vi "Modbus send and receive.vi"(6 "Modbus telegram":string, 7 "COM port":refnum<visa-resource-name>) -> (0 "Comms error":errorcluster, 1 "Device response":u8[](array[numeric]) format="%02x", 2 "Modbus exception code":T1 items=["None"=0, "Invalid function request"=1, "Invalid Modbus register address"=2, "Invalid / unauthorised data value"=3, "Device failure"=4, "Request accepted, wait"=5, "Drive busy"=6, "Request rejected"=7, "Memory parity error"=8, "Gateway path unavailable"=10, "Device failed to respond"=11], 3 "Checksum ok":bool)   [LabVIEW 2020]
doc: "Modbus RTU for Invertek drives. Paul Nathan 19-JUN-2022."
uses:
  ctls/Exception codes.ctl
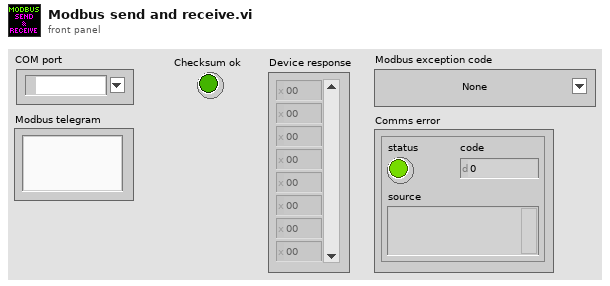
[diagram p1: front panel]
types:
  T1 = typedef "Exception codes.ctl" = u8
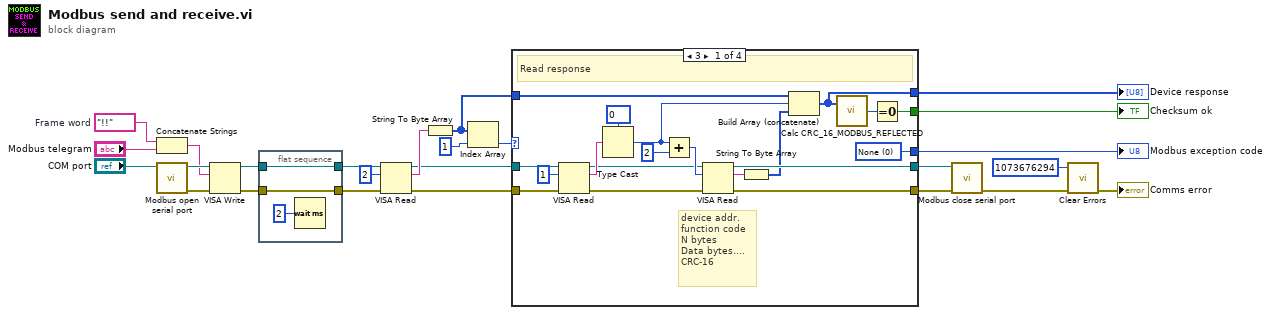
[diagram p0: block diagram]
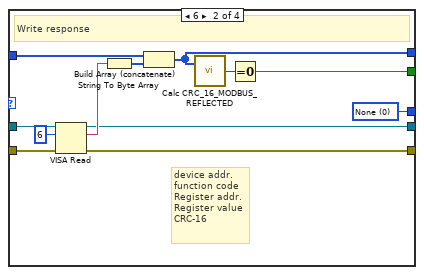
[diagram p2: hidden frame]
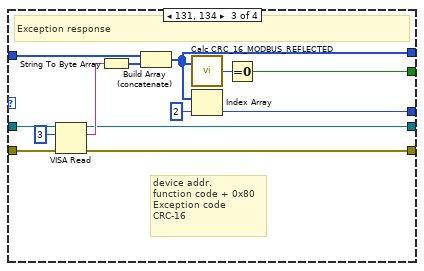
[diagram p3: hidden frame]
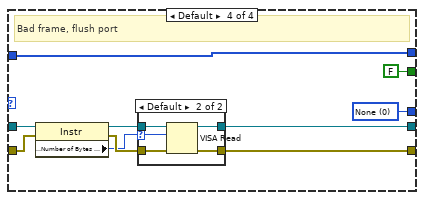
[diagram p4: hidden frame]
diagram:
  w1 = "!!"  # Frame word
  n1 = Concatenate Strings(w1, "Modbus telegram") -> (w2:string)
  n2 = call "Modbus open serial port.vi"("VISA resource name"="COM port") -> ("Error out"=w24:errorcluster, "VISA resource name out"=w25:refnum<visa-resource-name>)  [unwired: 9 in]
  n3 = VISA Write(VISA resource name=w25, write buffer=w2, error in (no error)=w24) -> (VISA resource name out=w7:refnum<visa-resource-name>, error out=w6:errorcluster)  [unwired: 1 out]
  n4 = flat-sequence {
    tunnel: w7 -> [w28]
    tunnel: w6 -> [w27]
    tunnel: [w28] -> w5
    tunnel: [w27] -> w4
    frame #0 {
      n5 = Wait (ms)(milliseconds to wait=u32 2) -> ()  [unwired: 1 out]
    }
  }
  n6 = VISA Read(VISA resource name=w5, byte count=u32 2, error in (no error)=w4) -> (VISA resource name out=w21:refnum<visa-resource-name>, read buffer=w22:string, error out=w20:errorcluster)  [unwired: 1 out]
  n7 = String To Byte Array(string=w22) -> (unsigned byte array=w16:u8[])
  n8 = Index Array(array=w16, index=1) -> (element=w17:u8)
  n9 = case shown="3" w17 {
    tunnel: w21 -> [w47 w59 w68 w82]
    tunnel: w20 -> [w46 w58 w67 w81]
    tunnel: [w37 w53 w64 w78] -> w19
    tunnel: [w33 w50 w65 FALSE] -> w13
    tunnel: [w32 w49 w62 w76] -> w12
    tunnel: w16 -> [w31 w56 w66 w76]
    tunnel: [w30 w52 w63 w77] -> w15
    tunnel: [w29 w48 w60 w74] -> w14
    frame 3 {
      w29 = T1 0 items=["None"=0, "Invalid request"=1, "Invalid Modbus register"=2, "Register value out of range"=3, "Device failure"=4, "Request accepted, wait"=5, "Drive busy"=6, "Request rejected"=7, "Memory parity error"=8, "Gateway path unavailable"=10, "Device failed to respond"=11] ("Modbus exception code")
      # "device addr.\nfunction code\nN bytes\nData bytes....\nCRC-16"
      # "Read response"
      n10 = VISA Read(VISA resource name=w47, byte count=u32 1, error in (no error)=w46) -> (VISA resource name out=w40:refnum<visa-resource-name>, read buffer=w44:string, error out=w39:errorcluster)  [unwired: 1 out]
      n11 = Type Cast(type=u8 0 ("index"), x=w44) -> (*(type *) &x=w36:u8)
      n12 = Add(x=w36, y=u32 2) -> (x+y=w41:u32)
      n13 = VISA Read(VISA resource name=w40, byte count=w41, error in (no error)=w39) -> (VISA resource name out=w37:refnum<visa-resource-name>, read buffer=w38:string, error out=w30:errorcluster)  [unwired: 1 out]
      n14 = String To Byte Array(string=w38) -> (unsigned byte array=w35:u8[])
      n15 = Build Array (concatenate)(w31, w36, w35) -> (w32:u8[])
      n16 = call "Calc CRC_16_MODBUS_REFLECTED.vi"("Data bytes"=w32) -> ("CRC_16-MODBUS"=w34:u16)  [unwired: 1 in]
      n17 = Equal To 0?(x=w34) -> (x = 0?=w33:bool)
    }
    frame 6 {
      w48 = T1 0 items=["None"=0, "Invalid request"=1, "Invalid Modbus register"=2, "Register value out of range"=3, "Device failure"=4, "Request accepted, wait"=5, "Drive busy"=6, "Request rejected"=7, "Memory parity error"=8, "Gateway path unavailable"=10, "Device failed to respond"=11] ("Modbus exception code")
      # "device addr.\nfunction code\nRegister addr.\nRegister value\nCRC-16"
      # "Write response"
      n18 = VISA Read(VISA resource name=w59, byte count=u32 6, error in (no error)=w58) -> (VISA resource name out=w53:refnum<visa-resource-name>, read buffer=w55:string, error out=w52:errorcluster)  [unwired: 1 out]
      n19 = String To Byte Array(string=w55) -> (unsigned byte array=w54:u8[])
      n20 = Build Array (concatenate)(w56, w54) -> (w49:u8[])
      n21 = call "Calc CRC_16_MODBUS_REFLECTED.vi"("Data bytes"=w49) -> ("CRC_16-MODBUS"=w51:u16)  [unwired: 1 in]
      n22 = Equal To 0?(x=w51) -> (x = 0?=w50:bool)
    }
    frame 131, 134 {
      # "device addr.\nfunction code + 0x80\nException code\nCRC-16"
      # "Exception response"
      n23 = VISA Read(VISA resource name=w68, byte count=u32 3, error in (no error)=w67) -> (VISA resource name out=w64:refnum<visa-resource-name>, read buffer=w72:string, error out=w63:errorcluster)  [unwired: 1 out]
      n24 = String To Byte Array(string=w72) -> (unsigned byte array=w71:u8[])
      n25 = Build Array (concatenate)(w66, w71) -> (w62:u8[])
      n26 = call "Calc CRC_16_MODBUS_REFLECTED.vi"("Data bytes"=w62) -> ("CRC_16-MODBUS"=w70:u16)  [unwired: 1 in]
      n27 = Index Array(array=w62, index=2) -> (element=w60:u8)
      n28 = Equal To 0?(x=w70) -> (x = 0?=w65:bool)
    }
    frame Default {
      w74 = T1 0 items=["None"=0, "Invalid request"=1, "Invalid Modbus register"=2, "Register value out of range"=3, "Device failure"=4, "Request accepted, wait"=5, "Drive busy"=6, "Request rejected"=7, "Memory parity error"=8, "Gateway path unavailable"=10, "Device failed to respond"=11] ("Modbus exception code")
      # "Bad frame, flush port"
      n29 = property class="Instr"(reference=w82, error in=w81) -> (reference out=w80:refnum<visa-resource-name>, error out=w79:errorcluster, "Serial Settings:Number of Bytes at Serial Port"=w73:u32)
      n30 = case shown="Default" w73 {
        selector: w73 -> [_ w85]
        tunnel: w80 -> [w84 w89]
        tunnel: w79 -> [w83 w88]
        tunnel: [w84 w87] -> w78
        tunnel: [w83 w86] -> w77
        frame 0 {
        }
        frame Default {
          n31 = VISA Read(VISA resource name=w89, byte count=w85, error in (no error)=w88) -> (VISA resource name out=w87:refnum<visa-resource-name>, error out=w86:errorcluster)  [unwired: 2 out]
        }
      }
    }
  }
  "Modbus exception code" <- w14
  "Checksum ok" <- w13
  "Device response" <- w12
  n32 = call "Modbus close serial port.vi"("Error in"=w15, "VISA resource name"=w19) -> ("Error out"=w9:errorcluster)  [unwired: 9 in]
  n33 = call <vilib>:"Clear Errors.vi"("error in (no error)"=w9, "specific error code to clear (0: all)"=1073676294) -> ("error out"=→"Comms error":errorcluster)  [unwired: 4 in, 1 out]
